vi "android_aceleração.vi"(11 "Dados Sensor":string) -> (3 "Aceleração":dbl)   [LabVIEW 2016]
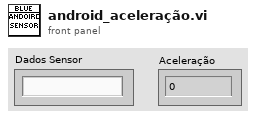
[diagram p1: front panel]
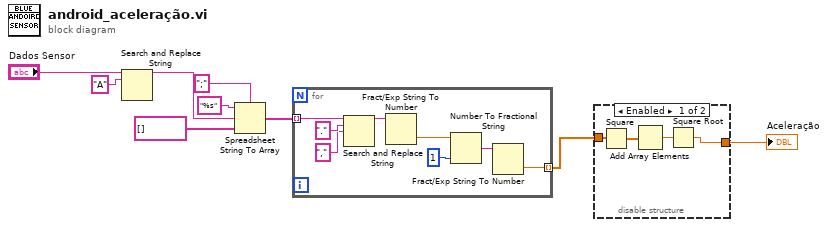
[diagram p0: block diagram]
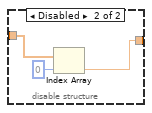
[diagram p2: hidden frame]
diagram:
  n1 = Search and Replace String(input string="Dados Sensor", search string="A") -> (result string=w6:string)  [unwired: 6 in, 3 out]
  n2 = Spreadsheet String To Array(delimiter (Tab)=";", format string="%s", spreadsheet string=w6, array type (2D Dbl)=string[] []) -> (array=w3:string[])
  n3 = for {
    tunnel: w3 -> [w17] mode=indexing
    tunnel: [w10] -> w2 mode=indexing
    n4 = Search and Replace String(input string=w17, search string=".", replace string="," ("replace string (\"\")")) -> (result string=w14:string)  [unwired: 5 in, 3 out]
    n5 = Fract/Exp String To Number(string=w14) -> (number=w13:dbl)  [unwired: 3 in, 1 out]
    n6 = Number To Fractional String(number=w13, precision (6)=i16 1) -> (F-format string=w11:string)  [unwired: 2 in]
    n7 = Fract/Exp String To Number(string=w11) -> (number=w10:dbl)  [unwired: 3 in, 1 out]
  }
  n8 = disable-structure shown="Enabled" {
    disable-tunnel: w2 -> [w20 w24]
    disable-tunnel: [w18 w22] -> w1
    frame Enabled {
      n9 = Square(x=w20) -> (x^2=w19:dbl[])
      n10 = Add Array Elements(numeric array=w19) -> (sum=w21:dbl)
      n11 = Square Root(x=w21) -> (sqrt(x)=w18:dbl)
    }
    frame Disabled {
      n12 = Index Array(array=w24, index=0) -> (element=w22:dbl)
    }
  }
  "Aceleração" <- w1
